vi "SetParam.vi"(8 "error in (no error)":errorcluster caption="entrée d'erreur (pas d'erreur)", 10 "coverage_error":cluster{"sample_weight":dbl[]}, 11 "Coverage_Error.lvclass":refnum<class "Coverage_Error.lvclass">) -> (0 "error out":errorcluster caption="sortie d'erreur", 3 "Coverage_Error.lvclass":refnum<class "Coverage_Error.lvclass">)   [LabVIEW 2020, in "Coverage_Error.lvclass"]
doc: "Set Parameters"
uses:
  Coverage_Error.lvclass
  Coverage_Error.lvclass/Coverage_Error.ctl
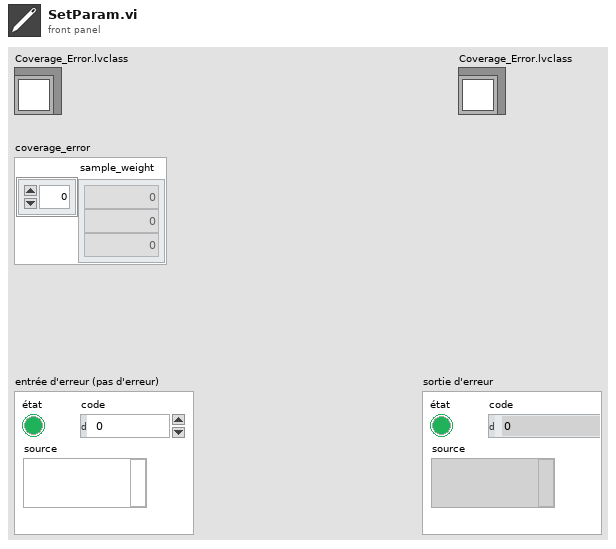
[diagram p1: front panel]
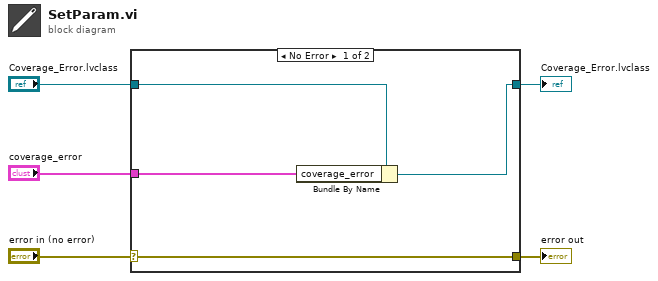
[diagram p0: block diagram]
diagram:
  n1 = case shown="No Error" "error in (no error)" {
    selector: "error in (no error)" -> [w9 w10]
    tunnel: [w9 w10] -> w4
    tunnel: [w7 w11] -> w2
    tunnel: "Coverage_Error.lvclass" -> [w8 w11]
    tunnel: "coverage_error" -> [w6 _]
    frame No Error {
      n2 = Bundle By Name(cluster=w8, "coverage_error"=w6) -> (w7:refnum<class "Coverage_Error.lvclass">)
    }
    frame Error {
    }
  }
  "error out" <- w4
  "Coverage_Error.lvclass" <- w2
